vi "icl_update_law.vi"() -> ()   [LabVIEW 2018]
panel:
  in  "queue":refnum<queue>
  in  "Array":refnum<k7>[](array[refnum])
  in  "y_sys_icl":dbl[][](array[numeric])
  in  "M":string
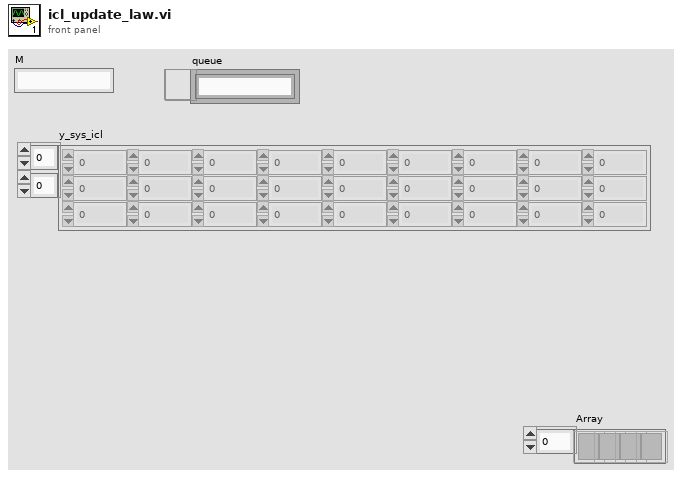
[diagram p1: front panel]
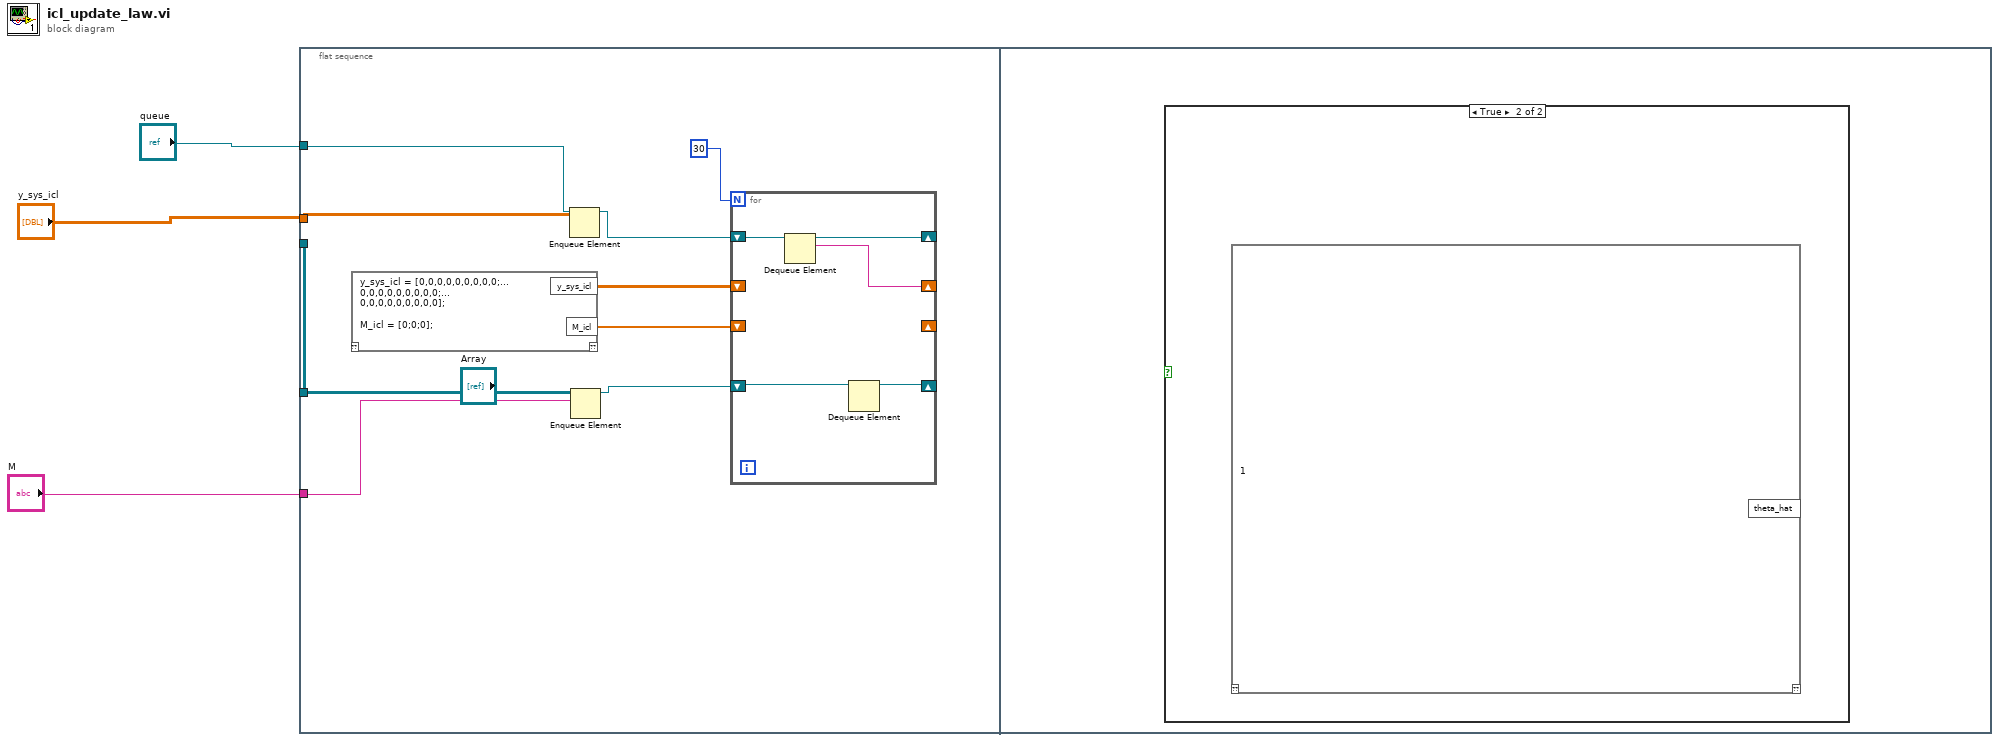
[diagram p0: block diagram]
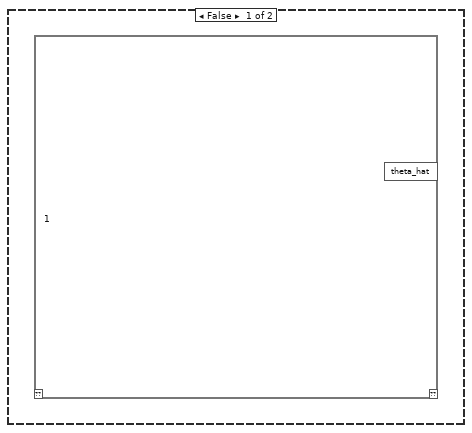
[diagram p2: hidden frame]
diagram:
  n1 = flat-sequence {
    tunnel: [w13] -> w2
    tunnel: "M" -> [w12]
    tunnel: "y_sys_icl" -> [w6]
    tunnel: w2 -> [_]
    tunnel: "queue" -> [w5]
    frame #0 {
      n2 = mathscript code="y_sys_icl = [0,0,0,0,0,0,0,0,0;...\n0,0,0,0,0,0,0,0,0;...\n0,0,0,0,0,0,0,0,0];\n\nM_icl = [0;0;0];"() -> ("y_sys_icl"=w8:dbl[][], "M_icl"=w7:dbl[])  [unwired: 1 in, 1 out]
      n3 = Enqueue Element(queue=w5, element=w6) -> (queue out=w10:refnum<queue>)  [unwired: 2 in, 2 out]
      n4 = Enqueue Element(queue=w13, element=w12) -> (queue out=w9:refnum<queue>)  [unwired: 2 in, 2 out]
      n5 = for {
        N: 30 -> [_]
        shift-right: [w17] -> _
        shift-left: w10 -> [w18]
        shift-right: [w15] -> _
        shift-left: w9 -> [w16]
        shift-right: [w14] -> _
        shift-left: w8 -> [_]
        shift-right: _ -> [_]
        shift-left: w7 -> [_]
        n6 = Dequeue Element(queue=w18) -> (queue out=w17:refnum<queue>, element=w14:string)  [unwired: 2 in, 2 out]
        n7 = Dequeue Element(queue=w16) -> (queue out=w15:refnum<queue>)  [unwired: 2 in, 3 out]
      }
    }
    frame #1 {
      n8 = case shown="True" {
        selector: _ -> [_ _]
        frame False {
          n9 = mathscript code="1"() -> ()  [unwired: 1 in, 2 out]
        }
        frame True {
          n10 = mathscript code="1"() -> ()  [unwired: 1 in, 2 out]
        }
      }
    }
  }
